vi "Obtain Request Events.vi"(8 "error in":errorcluster, 10 "Create New? (F)":bool) -> (0 "error out":errorcluster, 2 "Power Supply Request Events":T1)   [LabVIEW 2025, in "Power Supply.lvlib"]
doc: "This VI Obtains/Creates the Requests events that will be used for other modules to communicate with the module that owns this VI. These Requests events will be accessed only via Public API methods for this module.\n\n<b>NOTE</b>: The contents of this VI are automatically generated and modified by the <b>Tools > DQMH Consortium > DQMH</b> utilities. Consider using those utilities instead of making your own modifications to this VI.\n_____\nBased on DQMH Dev Tools: Project Template 7.1.2.1547."
uses:
  Power Supply.lvlib
  Request Events--cluster.ctl
  Stop Argument--cluster.ctl
  Show Panel Argument--cluster.ctl
  Hide Panel Argument--cluster.ctl
  Show Diagram Argument--cluster.ctl
  Get Module Execution Status Argument--cluster.ctl
  select child Argument--cluster.ctl
  Classes/hardware-selection.ctl
  select child (Reply Payload)--cluster.ctl
  read config Argument--cluster.ctl
  read config (Reply Payload)--cluster.ctl
  init device Argument--cluster.ctl
  init device (Reply Payload)--cluster.ctl
  close Argument--cluster.ctl
  close (Reply Payload)--cluster.ctl
  output Argument--cluster.ctl
  output (Reply Payload)--cluster.ctl
  set voltage Argument--cluster.ctl
  set voltage (Reply Payload)--cluster.ctl
  set current Argument--cluster.ctl
  set current (Reply Payload)--cluster.ctl
  read current Argument--cluster.ctl
  read current (Reply Payload)--cluster.ctl
  Controls/Numeric Current.ctl
  read voltage Argument--cluster.ctl
  read voltage (Reply Payload)--cluster.ctl
  Controls/Numeric Voltage.ctl
  read state Argument--cluster.ctl
  read state (Reply Payload)--cluster.ctl
  set all outputs Argument--cluster.ctl
  set all outputs (Reply Payload)--cluster.ctl
panel:
  # "NOTE: The contents of this VI are automatically generated and modified by the Tools > DQMH Consortium > DQMH utilities. Consider using those utilities instead of making your own modifications to this VI."
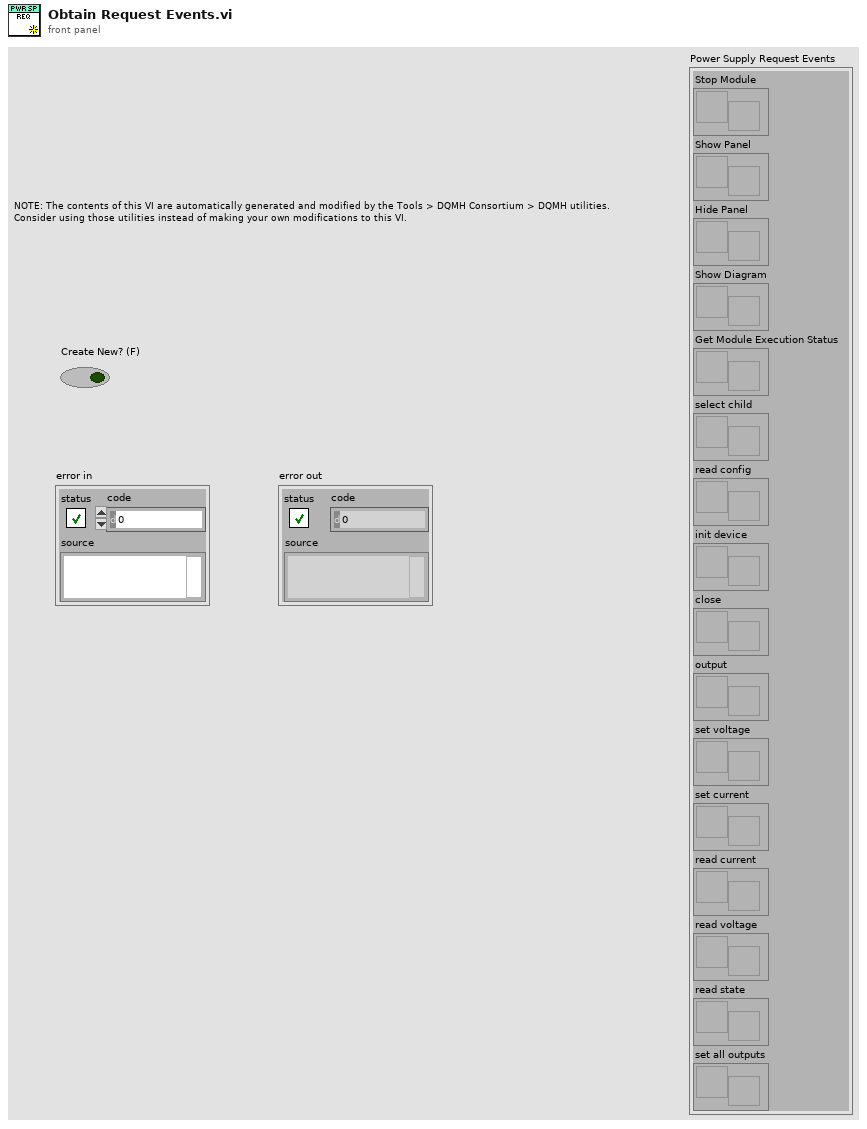
[diagram p1: front panel]
types:
  T1 = typedef "Power Supply.lvlib/Request Events--cluster.ctl" = cluster{"Stop Module":refnum<user-event>, "Show Panel":refnum<user-event>, "Hide Panel":refnum<user-event>, "Show Diagram":refnum<user-event>, "Get Module Execution Status":refnum<user-event>, "select child":refnum<user-event>, "read config":refnum<user-event>, "init device":refnum<user-event>, "close":refnum<user-event>, "output":refnum<user-event>, "set voltage":refnum<user-event>, "set current":refnum<user-event>, "read current":refnum<user-event>, "read voltage":refnum<user-event>, "read state":refnum<user-event>, "set all outputs":refnum<user-event>}
  T2 = typedef "Power Supply.lvlib/set all outputs Argument--cluster.ctl" = cluster{"Module ID":i32, "Voltage":dbl, "Current":dbl, "Output On/Off":bool, "Wait Notifier":refnum<notifier>, "wait for reply":bool}
  T3 = typedef "Power Supply.lvlib/read state Argument--cluster.ctl" = cluster{"Module ID":i32, "Wait Notifier":refnum<notifier>, "wait for reply":bool}
  T4 = typedef "Power Supply.lvlib/read voltage Argument--cluster.ctl" = cluster{"Module ID":i32, "Wait Notifier":refnum<notifier>, "wait for reply":bool}
  T5 = typedef "Power Supply.lvlib/read current Argument--cluster.ctl" = cluster{"Module ID":i32, "Wait Notifier":refnum<notifier>, "wait for reply":bool}
  T6 = typedef "Power Supply.lvlib/set current Argument--cluster.ctl" = cluster{"Module ID":i32, "Output Current":dbl, "Wait Notifier":refnum<notifier>, "wait for reply":bool}
  T7 = typedef "Power Supply.lvlib/set voltage Argument--cluster.ctl" = cluster{"Module ID":i32, "Output Voltage":dbl, "Wait Notifier":refnum<notifier>, "wait for reply":bool}
  T8 = typedef "Power Supply.lvlib/output Argument--cluster.ctl" = cluster{"Module ID":i32, "Output On/Off":bool, "Wait Notifier":refnum<notifier>, "wait for reply":bool}
  T9 = typedef "Power Supply.lvlib/close Argument--cluster.ctl" = cluster{"Module ID":i32, "Wait Notifier":refnum<notifier>, "wait for reply":bool}
  T10 = typedef "Power Supply.lvlib/init device Argument--cluster.ctl" = cluster{"Module ID":i32, "Variant":variant, "Wait Notifier":refnum<notifier>, "wait for reply":bool}
  T11 = typedef "Power Supply.lvlib/read config Argument--cluster.ctl" = cluster{"Module ID":i32, "config json file":path, "Wait Notifier":refnum<notifier>, "wait for reply":bool}
  T12 = typedef "Power Supply.lvlib/select child Argument--cluster.ctl" = cluster{"Module ID":i32, "Enum":T13, "Wait Notifier":refnum<notifier>, "wait for reply":bool}
  T13 = typedef "hardware-selection.ctl" = enum16{"Parent", "Simulation", "PSP-603"}
  T14 = typedef "Power Supply.lvlib/Get Module Execution Status Argument--cluster.ctl" = cluster{"Module ID":i32, "Running?":bool}
  T15 = typedef "Power Supply.lvlib/Show Diagram Argument--cluster.ctl" = cluster{"Module ID":i32, "Debug?":bool}
  T16 = typedef "Power Supply.lvlib/Show Panel Argument--cluster.ctl" = cluster{"Module ID":i32, "Show Panel?":bool}
  T17 = typedef "Power Supply.lvlib/Hide Panel Argument--cluster.ctl" = cluster{"Module ID":i32, "Hide Panel?":bool}
  T18 = typedef "Power Supply.lvlib/Stop Argument--cluster.ctl" = cluster{"Module ID":i32, "Origin":string, "Exit via Stop Module Req?":bool, "Wait for Module to stop?":bool}
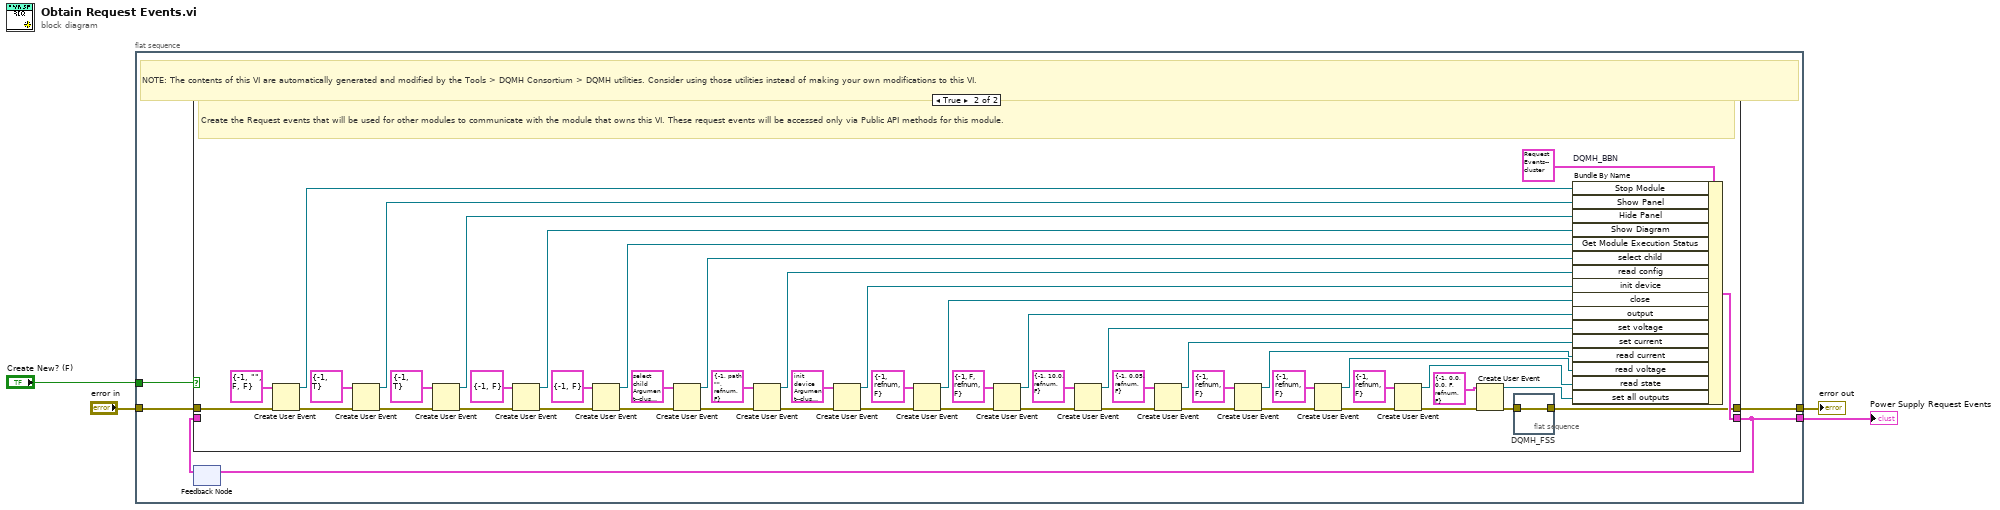
[diagram p0: block diagram]
diagram:
  n1 = flat-sequence {
    tunnel: [w9] -> w4
    tunnel: "error in" -> [w8]
    tunnel: [w6] -> w2
    tunnel: "Create New? (F)" -> [w5]
    frame #0 {
      # "NOTE: The contents of this VI are automatically generated and modified by the Tools > DQMH Consortium > DQMH utilities. Consider using those utilities instead of making your own modifications to this VI."
      n2 = feedback #1() -> (w7:T1)  [unwired: 1 in]
      n3 = case shown="True" w5 {
        tunnel: [w10 w51] -> w9
        tunnel: w8 -> [w10 w63]
        tunnel: [w11 w60] -> w6
        tunnel: w7 -> [w11 _]
        frame False {
        }
        frame True {
          # "Create the Request events that will be used for other modules to communicate with the module that owns this VI. These request events will be accessed only via Public API methods for this module."
          n4 = Create User Event(user event datatype=T18 {"Module ID"=-1, "Origin"="", "Exit via Stop Module Req?"=FALSE, "Wait for Module to stop?"=FALSE} ("Stop Argument"), error in=w63) -> (user event=w61:refnum<user-event>, error out=w58:errorcluster)
          n5 = Create User Event(user event datatype=T16 {"Module ID"=-1, "Show Panel?"=TRUE} ("Show Panel Argument"), error in=w58) -> (user event=w57:refnum<user-event>, error out=w55:errorcluster)
          n6 = Create User Event(user event datatype=T17 {"Module ID"=-1, "Hide Panel?"=TRUE} ("Hide Panel"), error in=w55) -> (user event=w54:refnum<user-event>, error out=w53:errorcluster)
          n7 = Create User Event(user event datatype=T15 {"Module ID"=-1, "Debug?"=FALSE} ("Show Diagram Argument"), error in=w53) -> (user event=w49:refnum<user-event>, error out=w50:errorcluster)
          n8 = Create User Event(user event datatype=T14 {"Module ID"=-1, "Running?"=FALSE} ("Get Module Execution Status Argument"), error in=w50) -> (user event=w46:refnum<user-event>, error out=w47:errorcluster)
          n9 = Create User Event(user event datatype=T12 {"Module ID"=-1, "Enum"=enum."PSP-603", "Wait Notifier"=refnum, "wait for reply"=FALSE} ("select child Argument"), error in=w47) -> (user event=w43:refnum<user-event>, error out=w44:errorcluster)
          n10 = Create User Event(user event datatype=T11 {"Module ID"=-1, "config json file"=path "", "Wait Notifier"=refnum, "wait for reply"=FALSE} ("read config Argument"), error in=w44) -> (user event=w40:refnum<user-event>, error out=w41:errorcluster)
          n11 = Create User Event(user event datatype=T10 {"Module ID"=-1, "Variant"=variant, "Wait Notifier"=refnum, "wait for reply"=FALSE} ("init device Argument"), error in=w41) -> (user event=w37:refnum<user-event>, error out=w38:errorcluster)
          n12 = Create User Event(user event datatype=T9 {"Module ID"=-1, "Wait Notifier"=refnum, "wait for reply"=FALSE} ("close Argument"), error in=w38) -> (user event=w34:refnum<user-event>, error out=w35:errorcluster)
          n13 = Create User Event(user event datatype=T8 {"Module ID"=-1, "Output On/Off"=FALSE, "Wait Notifier"=refnum, "wait for reply"=FALSE} ("output Argument"), error in=w35) -> (user event=w31:refnum<user-event>, error out=w32:errorcluster)
          n14 = Create User Event(user event datatype=T7 {"Module ID"=-1, "Output Voltage"=10.0, "Wait Notifier"=refnum, "wait for reply"=FALSE} ("set voltage Argument"), error in=w32) -> (user event=w28:refnum<user-event>, error out=w29:errorcluster)
          n15 = Create User Event(user event datatype=T6 {"Module ID"=-1, "Output Current"=0.05, "Wait Notifier"=refnum, "wait for reply"=FALSE} ("set current Argument"), error in=w29) -> (user event=w25:refnum<user-event>, error out=w26:errorcluster)
          n16 = Create User Event(user event datatype=T5 {"Module ID"=-1, "Wait Notifier"=refnum, "wait for reply"=FALSE} ("read current Argument"), error in=w26) -> (user event=w22:refnum<user-event>, error out=w23:errorcluster)
          n17 = Create User Event(user event datatype=T4 {"Module ID"=-1, "Wait Notifier"=refnum, "wait for reply"=FALSE} ("read voltage Argument"), error in=w23) -> (user event=w19:refnum<user-event>, error out=w20:errorcluster)
          n18 = Create User Event(user event datatype=T3 {"Module ID"=-1, "Wait Notifier"=refnum, "wait for reply"=FALSE} ("read state Argument"), error in=w20) -> (user event=w16:refnum<user-event>, error out=w17:errorcluster)
          n19 = Create User Event(user event datatype=T2 {"Module ID"=-1, "Voltage"=0.0, "Current"=0.0, "Output On/Off"=FALSE, "Wait Notifier"=refnum, "wait for reply"=FALSE} ("set all outputs Argument"), error in=w17) -> (user event=w13:refnum<user-event>, error out=w14:errorcluster)
          n20 = flat-sequence "DQMH_FSS" {
            tunnel: w14 -> [w64]
            tunnel: [w64] -> w51
            frame #0 {
            }
          }
          n21 = Bundle By Name "DQMH_BBN"(cluster=T1 {"Stop Module"=refnum, "Show Panel"=refnum, "Hide Panel"=refnum, "Show Diagram"=refnum, "Get Module Execution Status"=refnum, "select child"=refnum, "read config"=refnum, "init device"=refnum, "close"=refnum, "output"=refnum, "set voltage"=refnum, "set current"=refnum, "read current"=refnum, "read voltage"=refnum, "read state"=refnum, "set all outputs"=refnum} ("output cluster"), "Stop Module"=w61, "Show Panel"=w57, "Hide Panel"=w54, "Show Diagram"=w49, "Get Module Execution Status"=w46, "select child"=w43, "read config"=w40, "init device"=w37, "close"=w34, "output"=w31, "set voltage"=w28, "set current"=w25, "read current"=w22, "read voltage"=w19, "read state"=w16, "set all outputs"=w13) -> (w60:T1)
        }
      }
      n22 = feedback-in #1(w6) -> ()
    }
  }
  "Power Supply Request Events" <- w2
  "error out" <- w4
